vi "game.vi"(1 "Cluster 2":T1) -> (0 "x = y?":bool)   [LabVIEW 2014]
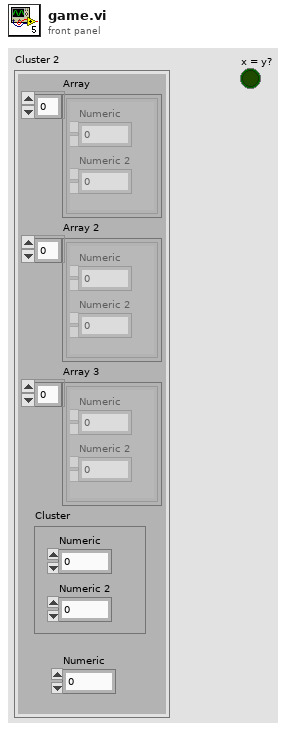
[diagram p1: front panel]
types:
  T1 = cluster{"Array":cluster{"Numeric":dbl, "Numeric 2":dbl}[], "Array 2":cluster{"Numeric":dbl, "Numeric 2":dbl}[], "Array 3":cluster{"Numeric":dbl, "Numeric 2":dbl}[], "Cluster":cluster{"Numeric":dbl, "Numeric 2":dbl}, "Numeric":dbl}
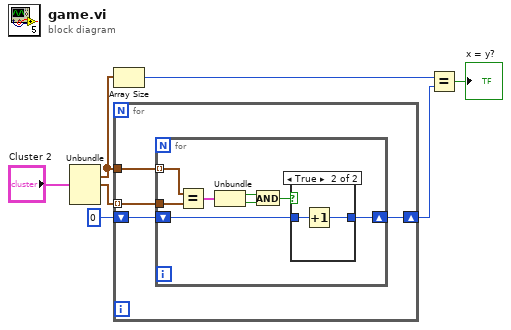
[diagram p0: block diagram]
diagram:
  n1 = Unbundle("Cluster 2") -> ("Array 2"=w1:cluster{"Numeric":dbl, "Numeric 2":dbl}[], "Array 3"=w2:cluster{"Numeric":dbl, "Numeric 2":dbl}[])  [unwired: 3 out]
  n2 = Array Size(array=w1) -> (size(s)=w5:i32)
  n3 = for {
    tunnel: w1 -> [w11]
    tunnel: w2 -> [w10] mode=indexing
    shift-right: [w8] -> w6
    shift-left: 0 -> [w9]
    n4 = for {
      tunnel: w11 -> [w18] mode=indexing
      tunnel: w10 -> [w17]
      shift-right: [w12] -> w8
      shift-left: w9 -> [w13]
      n5 = Equal?(x=w18, y=w17) -> (x = y?=w19:cluster{"Numeric":bool, "Numeric 2":bool})
      n6 = Unbundle(w19) -> ("Numeric"=w16:bool, "Numeric 2"=w15:bool)
      n7 = And(x=w16, y=w15) -> (x .and. y?=w14:bool)
      n8 = case shown="True" w14 {
        tunnel: w13 -> [w20 w22]
        tunnel: [w20 w21] -> w12
        frame False {
        }
        frame True {
          n9 = Increment(x=w22) -> (x+1=w21:i32)
        }
      }
    }
  }
  n10 = Equal?(x=w5, y=w6) -> (x = y?=→"x = y?":bool)
